vi "CanStatusShow.vi"(10 "DevIndex":u32, 11 "DevType":u16) -> ()   [LabVIEW 2011]
panel:
  in  "OK":bool
  out "regTECounter":u8 caption="CAN控制器发送错误寄存器：" format="0x%02x"
  out "regRECounter":u8 caption="CAN控制器接收错误寄存器：" format="0x%02x"
  out "regEWLimit":u8 caption="CAN控制器错误警告限制寄存器：" format="0x%02x"
  out "regECCapture":u8 caption="CAN控制器错误寄存器：" format="0x%02x"
  out "regALCapture":u8 caption="CAN控制器仲裁丢失寄存器：" format="0x%02x"
  out "regStatus":u8 caption="CAN控制器状态寄存器：" format="0x%02x"
  out "regMode":u8 caption="CAN控制器模式寄存器：" format="0x%02x"
  out "ErrInterrupt":u8 caption="中断记录：" format="0x%02x"
  in  "Update":bool
  in  "udtTime":i32=1 min=1 max=100 format="%d 秒"
  in  "Auto":bool
  in  "channel":enum16{"通道1", "通道2"}(ring) caption="CAN通道"
  # "寄存器信息"
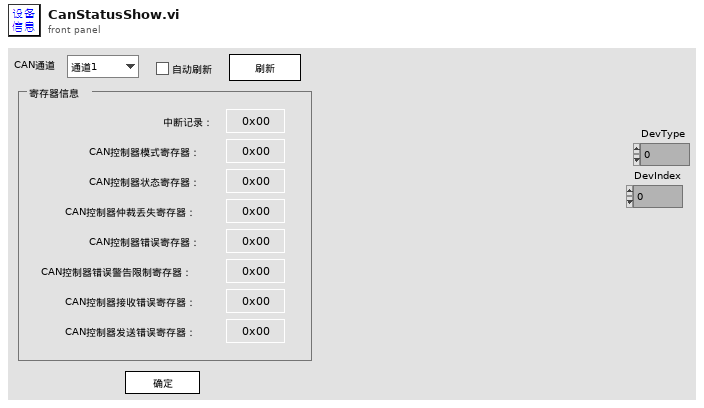
[diagram p1: front panel]
types:
  T1 = cluster{"ErrInterrupt":u8, "regMode":u8, "regStatus":u8, "regALCapture":u8, "regECCapture":u8, "regEWLimit":u8, "regRECounter":u8, "regTECounter":u8, "Reserved":u32}
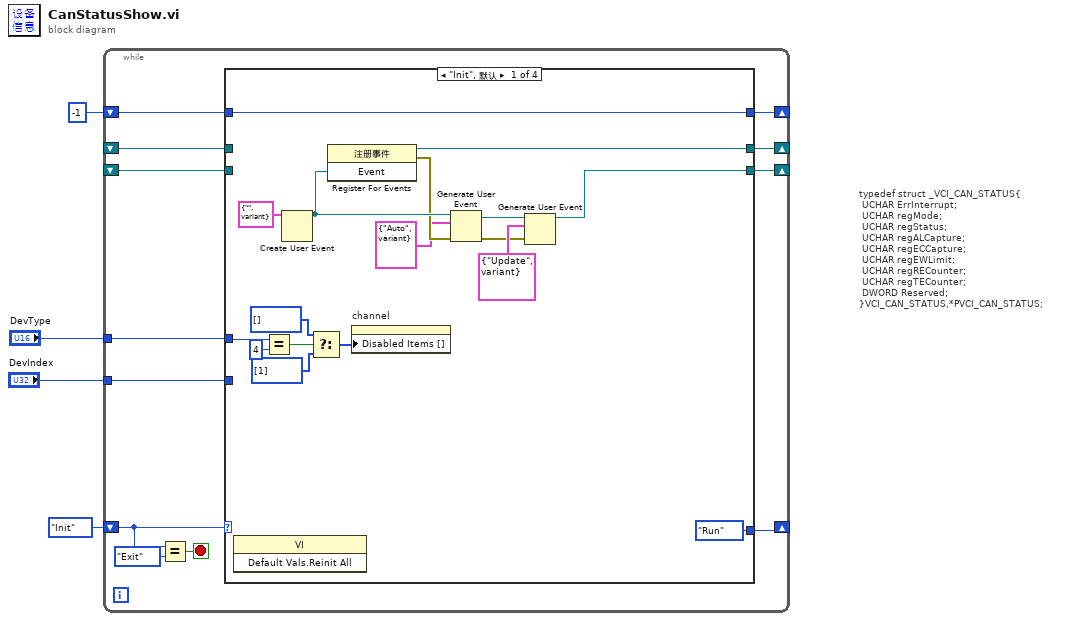
[diagram p0: block diagram]
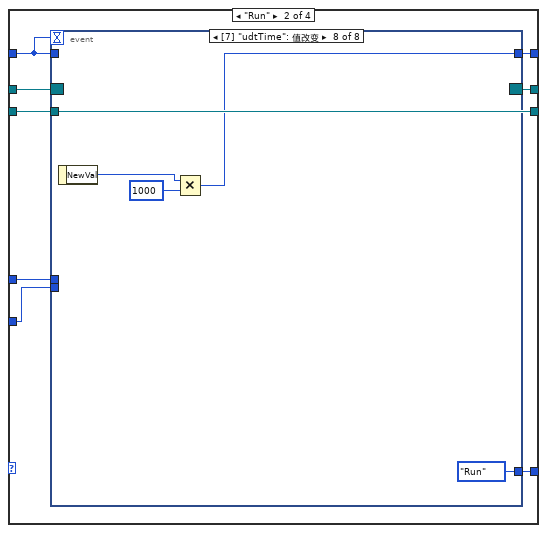
[diagram p2: hidden frame]
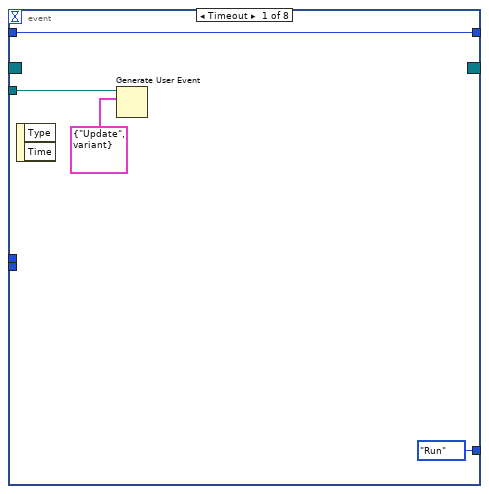
[diagram p3: hidden frame]
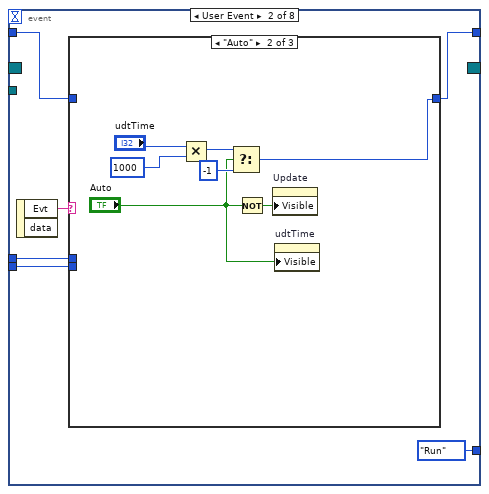
[diagram p4: hidden frame]
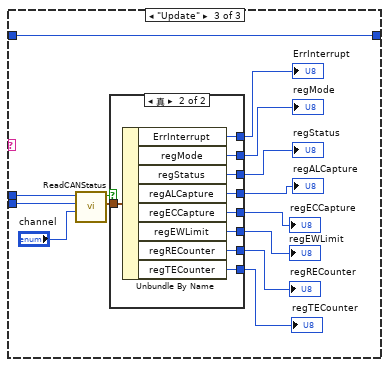
[diagram p6: hidden frame]
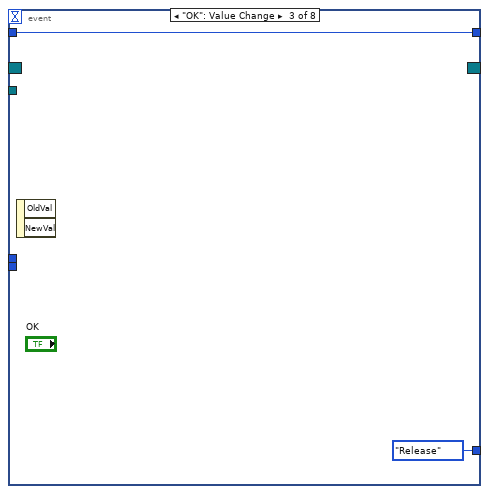
[diagram p8: hidden frame]
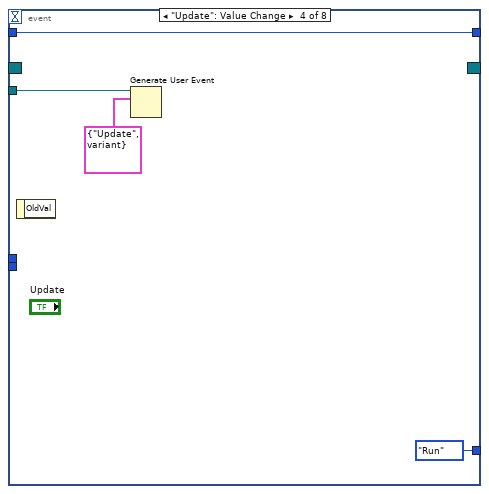
[diagram p9: hidden frame]
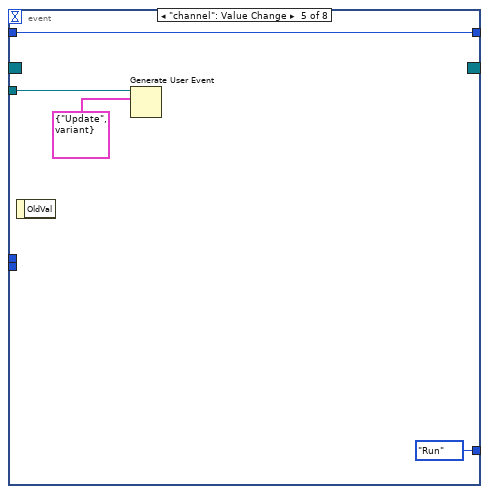
[diagram p10: hidden frame]
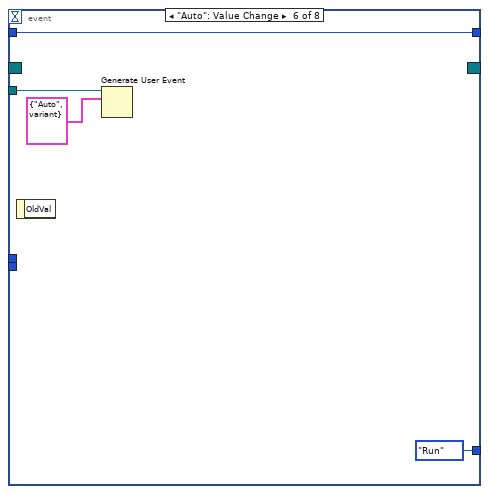
[diagram p11: hidden frame]
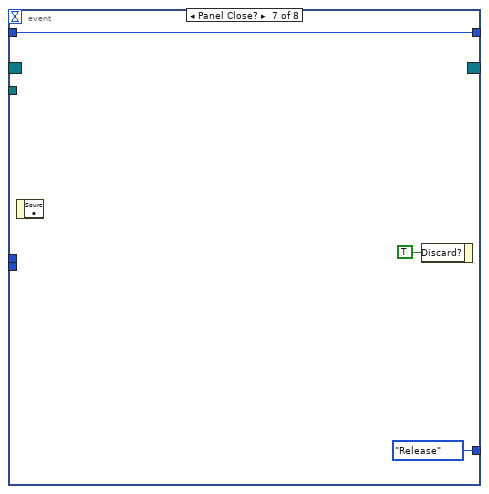
[diagram p12: hidden frame]
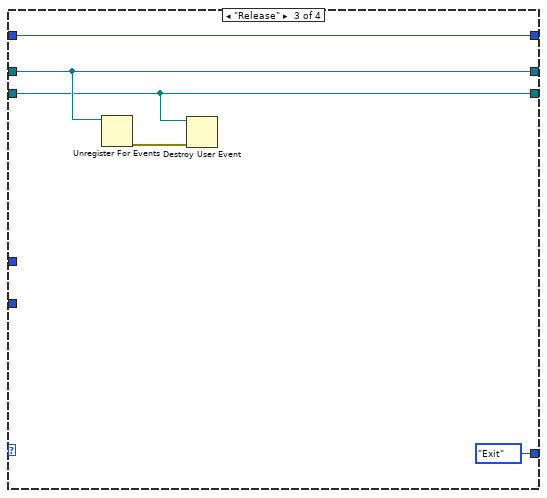
[diagram p13: hidden frame]
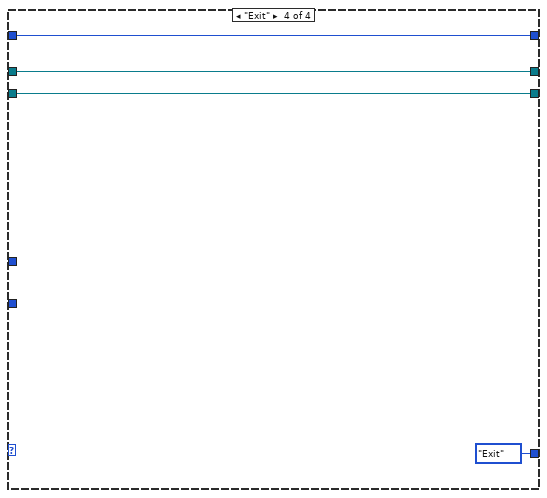
[diagram p14: hidden frame]
diagram:
  # "typedef struct _VCI_CAN_STATUS{\n\tUCHAR\tErrInterrupt;\n\tUCHAR\tregMode;\n\tUCHAR\tregStatus;\n\tUCHAR\tregALCapture;\n\tUCHAR\tregECCapture; \n\tUCHAR\tregEWLimit;\n\tUCHAR\tregRECounter; \n\tUCHAR\tregTECounter;\n\tDWORD\tReserved;\n}VCI_CAN_STATUS,*PVCI_CAN_STATUS;"
  n1 = while {
    shift-right: [w13] -> _
    shift-left: enum16{"Init", "Run", "Release", "Exit"}."Init" -> [w16]
    shift-right: [w12] -> _
    shift-left: _ -> [w11]
    tunnel: "DevType" -> [w10]
    tunnel: "DevIndex" -> [w9]
    shift-right: [w8] -> _
    shift-left: _ -> [w7]
    shift-right: [w5] -> _
    shift-left: -1 -> [w6]
    stop <- w14 stop-if-true
    n2 = Equal?(x=w16, y=enum16{"Init", "Run", "Release", "Exit"}."Exit") -> (x = y?=w14:bool)
    n3 = case shown="\"Init\", 默认" w16 {
      tunnel: [enum16{"Init", "Run", "Release", "Exit"}."Run" w41 enum16{"Init", "Run", "Release", "Exit"}."Exit" enum16{"Init", "Run", "Release", "Exit"}."Exit"] -> w13
      tunnel: [w31 w39 w107 w112] -> w12
      tunnel: w11 -> [_ w40 w107 w112]
      tunnel: w10 -> [w27 w35 _ _]
      tunnel: w9 -> [_ w34 _ _]
      tunnel: [w18 w38 w106 w111] -> w8
      tunnel: w7 -> [_ w38 w106 w111]
      tunnel: w6 -> [w17 w37 w108 w110]
      tunnel: [w17 w36 w108 w110] -> w5
      frame "Init", Default {
        n4 = invoke class="VI" method="Default Vals.Reinit All"() -> ()  [unwired: 3 in, 3 out]
        n5 = Equal?(x=w27, y=u16 4) -> (x = y?=w25:bool)
        n6 = Create User Event(user event datatype=cluster{"Evt":string, "data":variant} {"Evt"="", "data"=variant} ("Event")) -> (user event=w30:refnum<user-event>)  [unwired: 1 in, 1 out]
        n7 = Select(t=i32[] [] ("禁用项[]"), s=w25, f=i32[] [1] ("禁用项[]")) -> (s? t:f=w22:i32[])
        n8 = register-events(w30) -> (reference out=w31:refnum<event-registration>, error out=w29:errorcluster)  [unwired: 2 in]
        n9 = property on="channel" class="Enum (严格)"("Disabled Items []"=w22) -> ()  [unwired: 2 in, 2 out]
        n10 = Generate User Event(user event=w30, event data cluster=cluster{"Evt":string, "data":variant} {"Evt"="Auto", "data"=variant} ("事件数据"), error in=w29) -> (user event out=w20:refnum<user-event>, error out=w19:errorcluster)
        n11 = Generate User Event(user event=w20, event data cluster=cluster{"Evt":string, "data":variant} {"Evt"="Update", "data"=variant} ("事件数据"), error in=w19) -> (user event out=w18:refnum<user-event>)  [unwired: 1 out]
      }
      frame "Run" {
        n12 = event shown="[7] \"udtTime\": 值改变" {
          selector: w40 -> [_ _ _ _ _ _ _ _]
          dyn-events: [_ _ _ _ _ _ _ _] -> w39
          timeout: w37 -> [_ _ _ _ _ _ _ _]
          tunnel: [enum16{"Init", "Run", "Release", "Exit"}."Run" enum16{"Init", "Run", "Release", "Exit"}."Run" enum16{"Init", "Run", "Release", "Exit"}."Release" enum16{"Init", "Run", "Release", "Exit"}."Run" enum16{"Init", "Run", "Release", "Exit"}."Run" enum16{"Init", "Run", "Release", "Exit"}."Run" enum16{"Init", "Run", "Release", "Exit"}."Release" enum16{"Init", "Run", "Release", "Exit"}."Run"] -> w41
          tunnel: w38 -> [w42 _ _ w85 w89 w95 _ _]
          tunnel: w37 -> [w44 w49 w83 w87 w91 w94 w97 _]
          tunnel: [w44 w48 w83 w87 w91 w94 w97 w100] -> w36
          tunnel: w35 -> [_ w47 _ _ _ _ _ _]
          tunnel: w34 -> [_ w46 _ _ _ _ _ _]
          event Timeout {
            n13 = event-data() -> ()  [unwired: 1 in, 2 out]
            n14 = Generate User Event(user event=w42, event data cluster=cluster{"Evt":string, "data":variant} {"Evt"="Update", "data"=variant} ("事件数据")) -> ()  [unwired: 1 in, 2 out]
          }
          event User Event {
            n15 = event-data() -> ("Evt"=w50:string)  [unwired: 1 in, 1 out]
            n16 = case shown="\"Auto\"" w50 {
              tunnel: w49 -> [w52 _ w73]
              tunnel: [w52 w56 w73] -> w48
              tunnel: w47 -> [_ _ w72]
              tunnel: w46 -> [_ _ w71]
              frame "假", Default {
              }
              frame "Auto" {
                n17 = Multiply(x="udtTime", y=1000) -> (x*y=w57:i32)
                n18 = Select(t=w57, s="Auto", f=-1) -> (s? t:f=w56:i32)
                n19 = Not(x="Auto") -> (.not. x?=w54:bool)
                n20 = property on="Update" class="Bool"("Visible"=w54) -> ()  [unwired: 2 in, 2 out]
                n21 = property on="udtTime" class="DigNum (严格)"("Visible"="Auto") -> ()  [unwired: 2 in, 2 out]
              }
              frame "Update" {
                n22 = call "ReadCANStatus.vi"("CANInd"="channel", "DeciceInd"=w71, "DeviceType"=w72) -> ("VCI_CAN_STATUS"=w68:T1, "Valid"=w69:bool)  [unwired: 6 in, 1 out]
                n23 = case shown="真" w69 {
                  tunnel: w68 -> [_ w82]
                  tunnel: [_ w81] -> w67
                  tunnel: [_ w80] -> w66
                  tunnel: [_ w79] -> w65
                  tunnel: [_ w78] -> w64
                  tunnel: [_ w77] -> w63
                  tunnel: [_ w76] -> w62
                  tunnel: [_ w75] -> w61
                  tunnel: [_ w74] -> w60
                  frame False {
                  }
                  frame True {
                    n24 = Unbundle By Name(w82) -> ("ErrInterrupt"=w81:u8, "regMode"=w80:u8, "regStatus"=w79:u8, "regALCapture"=w78:u8, "regECCapture"=w77:u8, "regEWLimit"=w76:u8, "regRECounter"=w75:u8, "regTECounter"=w74:u8)
                  }
                }
                "ErrInterrupt" <- w67
                "regMode" <- w66
                "regStatus" <- w65
                "regALCapture" <- w64
                "regECCapture" <- w63
                "regEWLimit" <- w62
                "regRECounter" <- w61
                "regTECounter" <- w60
              }
            }
          }
          event "OK": Value Change {
            n25 = event-data() -> ()  [unwired: 1 in, 2 out]
          }
          event "Update": Value Change {
            n26 = event-data() -> ()  [unwired: 1 in, 1 out]
            n27 = Generate User Event(user event=w85, event data cluster=cluster{"Evt":string, "data":variant} {"Evt"="Update", "data"=variant} ("事件数据")) -> ()  [unwired: 1 in, 2 out]
          }
          event "channel": Value Change {
            n28 = event-data() -> ()  [unwired: 1 in, 1 out]
            n29 = Generate User Event(user event=w89, event data cluster=cluster{"Evt":string, "data":variant} {"Evt"="Update", "data"=variant} ("事件数据")) -> ()  [unwired: 1 in, 2 out]
          }
          event "Auto": Value Change {
            n30 = event-data() -> ()  [unwired: 1 in, 1 out]
            n31 = Generate User Event(user event=w95, event data cluster=cluster{"Evt":string, "data":variant} {"Evt"="Auto", "data"=variant} ("事件数据")) -> ()  [unwired: 1 in, 2 out]
          }
          event Panel Close? {
            n32 = event-data() -> ()  [unwired: 1 in, 1 out]
            n33 = event-data("Discard?"=TRUE ("放弃？")) -> ()  [unwired: 1 in, 1 out]
          }
          event "udtTime": Value Change {
            n34 = event-data() -> ("NewVal"=w102:i32)  [unwired: 1 in]
            n35 = Multiply(x=w102, y=1000) -> (x*y=w100:i32)
          }
        }
      }
      frame "Release" {
        n36 = Unregister For Events(event registration refnum=w107) -> (error out=w105:errorcluster)  [unwired: 1 in]
        n37 = Destroy User Event(user event=w106, error in=w105) -> ()  [unwired: 1 out]
      }
      frame "Exit" {
      }
    }
  }
